vi "Append VI Hierarchy to Report (path).vi"(0 "report in":refnum<class "NI_report.lvclass">, 2 "image format (jpeg)":enum32{"PNG", "JPEG", "GIF"}(ring)=enum."JPEG", 5 "VI":path, 7 "alignment (default)":T2, 11 "error in (no error)":errorcluster, 12 "MS Office parameters":T1) -> (4 "report out":refnum<class "NI_report.lvclass">, 6 "VI path out":path, 8 "start out (Word)":i32, 10 "end out (Word)":i32, 15 "error out":errorcluster)   [LabVIEW 2017, in "NI_ReportGenerationCore.lvlib"]
doc: "Appends the hierarchy of the VI you specify in <B>VI</B> to a report. Wire data to the <B>VI</B> input to determine the polymorphic instance to use or manually select the instance."
uses:
  <vilib>/Utility/NIReport.llb/NI_ReportGenerationCore.lvlib
  <vilib>/Utility/NIReport.llb/NI_report.lvclass
  <vilib>/Utility/NIReport.llb/HTML Report Image Alignment.ctl
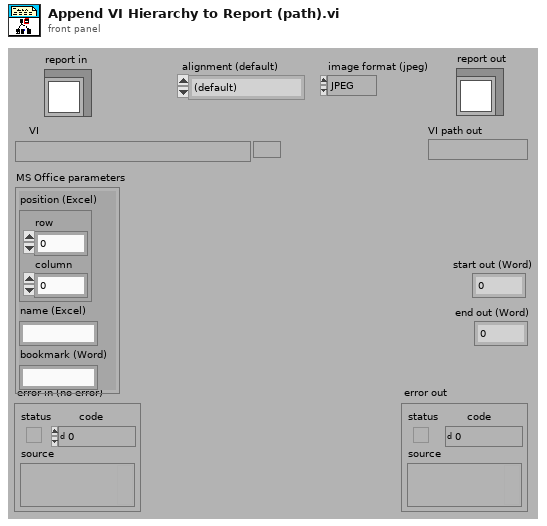
[diagram p1: front panel]
types:
  T1 = cluster{"position (Excel)":cluster{"row":i32, "column":i32}, "name (Excel)":string, "bookmark (Word)":string}
  T2 = typedef "NI_ReportGenerationCore.lvlib/HTML Report Image Alignment.ctl" = enum16{"(default)", "LEFT", "RIGHT", "TOP", "TEXTTOP", "MIDDLE", "ABSMIDDLE", "BASELINE", "BOTTOM", "ABSBOTTOM"}
  T3 = enum32{"invalid app kind", "Development System", "Run Time System", "Student Edition", "Embedded LabVIEW", "Evaluation", "Custom"}
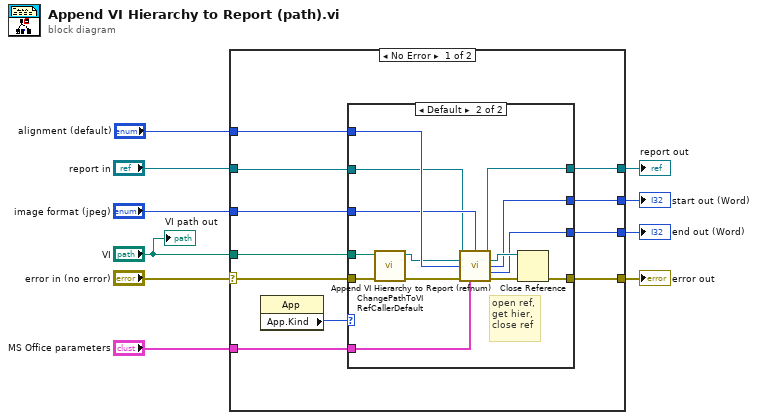
[diagram p0: block diagram]
diagram:
  n1 = case shown="No Error" "error in (no error)" {
    selector: "error in (no error)" -> [w21 w39]
    tunnel: [w16 w39] -> w9
    tunnel: [w14 w38] -> w7
    tunnel: "report in" -> [w15 w38]
    tunnel: "VI" -> [w20 _]
    tunnel: "image format (jpeg)" -> [w17 _]
    tunnel: "MS Office parameters" -> [w19 _]
    tunnel: "alignment (default)" -> [w18 _]
    tunnel: [w13 _] -> w2
    tunnel: [w12 _] -> w1
    frame No Error {
      n2 = property class="App"() -> ("App.Kind"=w11:T3)  [unwired: 2 in, 2 out]
      n3 = case shown="Default" w11 {
        tunnel: w21 -> [w22 w37]
        tunnel: w20 -> [_ w35]
        tunnel: w19 -> [_ w34]
        tunnel: w18 -> [_ w33]
        tunnel: w17 -> [_ w32]
        tunnel: [w22 w30] -> w16
        tunnel: w15 -> [w23 w27]
        tunnel: [w23 w26] -> w14
        tunnel: [_ w25] -> w13
        tunnel: [_ w24] -> w12
        frame "Run Time System" {
          # "Do not try to append\nif running in an\nexecutable"
        }
        frame Default {
          # "open ref,\nget hier,\nclose ref"
          n4 = call <vilib>:"ChangePathToVIRefCallerDefault.vi"("error in (no error)"=w37, "VI path"=w35) -> ("error out"=w36:errorcluster, "VI reference"=w28:refnum<vi>)  [unwired: 4 in]
          n5 = call <vilib>:"Append VI Hierarchy to Report (refnum).vi"("report in"=w27, "image format (jpeg)"=w32, "VI"=w28, "alignment (default)"=w33, "error in (no error)"=w36, "MS Office parameters"=w34) -> ("report out"=w26:refnum<class "NI_report.lvclass">, "VI out"=w29:refnum<vi>, "start out (Word)"=w25:i32, "end out (Word)"=w24:i32, "error out"=w31:errorcluster)  [unwired: 5 in]
          n6 = Close Reference(reference=w29, error in (no error)=w31) -> (error out=w30:errorcluster)
        }
      }
    }
    frame Error {
    }
  }
  "error out" <- w9
  "report out" <- w7
  "start out (Word)" <- w2
  "end out (Word)" <- w1
  "VI path out" <- "VI"
